vi "Write types.vi"(8 "error in (no error)":errorcluster, 10 "types":T1[](array[typedef]), 11 "bt_WaitOn_Queue in":refnum<class "bt_WaitOn_Queue.lvclass">) -> (0 "error out":errorcluster, 3 "bt_WaitOn_Queue out":refnum<class "bt_WaitOn_Queue.lvclass">)   [LabVIEW 2021, in "BT.lvlib" / "bt_WaitOn_Queue.lvclass"]
uses:
  bt_WaitOn_Queue.lvclass
  bt_WaitOn_Queue.lvclass/bt_WaitOn_Queue.ctl
  <vilib>/Utility/Data Type/Type Definitions/Data Type.ctl
  <vilib>/Utility/Data Type/NI_Data Type.lvlib
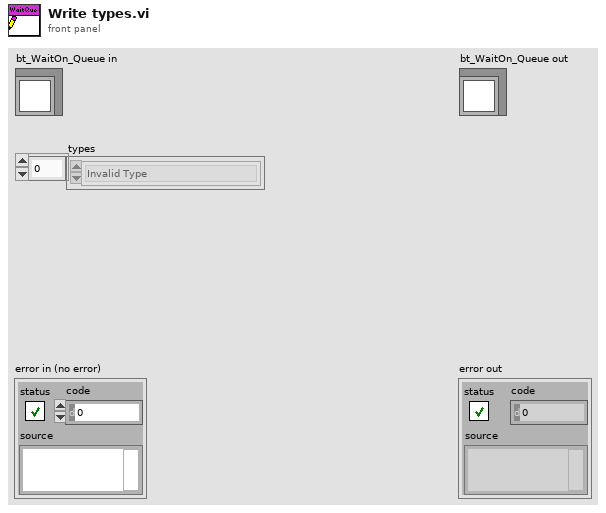
[diagram p1: front panel]
types:
  T1 = typedef "NI_Data Type.lvlib/Data Type.ctl" = enum8{"Invalid Type", "Void", "I8", "I16", "I32", "I64", "U8", "U16", "U32", "U64", "Single Float", "Double Float", "Extended Float", "Single Complex", "Double Complex", "Extended Complex", "Enum U8", "Enum U16", "Enum U32", "Enum U64", "Single Float With Unit", "Double Float With Unit", "Extended Float With Unit", "Single Complex with Unit", "Double Complex with Unit", "Extended Complex with Unit", "Boolean", "String", "Path", "Picture", "Tag", "Array", "Cluster", "Variant", "LV Variant", "Waveform", "Timestamp", "Digital Waveform", "Digital Data", "ExpressData", "Refnum", "External Data", "VI", "Poly VI", "LabVIEW Class Instance", "Fixed Point", "Set Collection", "Map Collection"}
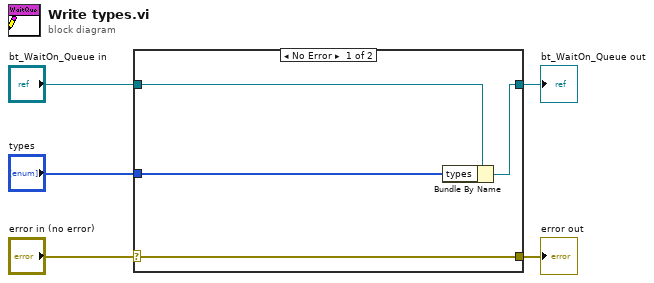
[diagram p0: block diagram]
diagram:
  n1 = case shown="No Error" "error in (no error)" {
    selector: "error in (no error)" -> [w9 w10]
    tunnel: [w9 w10] -> w4
    tunnel: [w7 w11] -> w2
    tunnel: "bt_WaitOn_Queue in" -> [w8 w11]
    tunnel: "types" -> [w6 _]
    frame No Error {
      n2 = Bundle By Name(cluster=w8, "types"=w6) -> (w7:refnum<class "bt_WaitOn_Queue.lvclass">)
    }
    frame Error {
    }
  }
  "error out" <- w4
  "bt_WaitOn_Queue out" <- w2
